vi "TestingBugFix.vi"() -> ()   [LabVIEW 2010]
uses:
  cm2nm_sample_set.ctl
  cm2nm_coordinate_information_v2.ctl
panel:
  out "Current Session Information":T1={"CollectionOfPoints"=[{"MetaDataFile"=path "", "X"=6.4684, "Y"=5.668, "Group"=0, "Z"=9.9998, "Rotation"=0.0, "Fiducial"=TRUE, "Magnification"=0.0, "Working_Distance"=0.0, "Notes"="Enter notes about this spot here.", "Location Name/ID"="Fid1", "OtherRelatedDataFiles"=[], "Available"=FALSE}, {"MetaDataFile"=path "", "X"=6.7812, "Y"=-3.8607, "Group"=0, "Z"=9.9998, "Rotation"=0.0, "Fiducial"=TRUE, "Magnification"=0.0, "Working_Distance"=0.0, "Notes"="Enter notes about this spot here.", "Location Name/ID"="Fid2", "OtherRelatedDataFiles"=[], "Available"=FALSE}, {"MetaDataFile"=path "", "X"=-3.5669, "Y"=-7.5774, "Group"=0, "Z"=9.9998, "Rotation"=0.0, "Fiducial"=TRUE, "Magnification"=0.0, "Working_Distance"=0.0, "Notes"="Enter notes about this spot here.", "Location Name/ID"="Fid3", "OtherRelatedDataFiles"=[], "Available"=FALSE}, {"MetaDataFile"=path "", "X"=4.04214894226502, "Y"=-0.78740272281952, "Group"=0, "Z"=9.9998, "Rotation"=0.0, "Fiducial"=FALSE, "Magnification"=0.0, "Working_Distance"=0.0, "Notes"="This is what we saw at the calculated coordinates for POI1. It's obviously not right! Look at images for calculated POI1.", "Location Name/ID"="POI1-calculated", "OtherRelatedDataFiles"=[], "Available"=FALSE}, {"MetaDataFile"=path "", "X"=0.4122, "Y"=-2.0241, "Group"=0, "Z"=0.0, "Rotation"=0.0, "Fiducial"=FALSE, "Magnification"=0.0, "Working_Distance"=0.0, "Notes"="These are the current coordinates of the real point", "Location Name/ID"="Actual POI1", "OtherRelatedDataFiles"=[], "Available"=FALSE}, {"MetaDataFile"=path "", "X"=0.41202447787402247, "Y"=-2.022580250416809, "Group"=20, "Z"=9.9998, "Rotation"=0.0, "Fiducial"=FALSE, "Magnification"=0.0, "Working_Distance"=0.0, "Notes"="Enter notes about this spot here.", "Location Name/ID"="POI1", "OtherRelatedDataFiles"=[], "Available"=FALSE}, {"MetaDataFile"=path "", "X"=-5.057894089920385, "Y"=8.260873627058263, "Group"=20, "Z"=9.9998, "Rotation"=0.0, "Fiducial"=TRUE, "Magnification"=0.0, "Working_Distance"=0.0, "Notes"="Enter notes about this spot here.", "Location Name/ID"="Fid5", "OtherRelatedDataFiles"=[], "Available"=FALSE}, {"MetaDataFile"=path "", "X"=-9.447460259107727, "Y"=0.8548991441777762, "Group"=20, "Z"=9.9998, "Rotation"=0.0, "Fiducial"=TRUE, "Magnification"=0.0, "Working_Distance"=0.0, "Notes"="Enter notes about this spot here.", "Location Name/ID"="Fid4", "OtherRelatedDataFiles"=[], "Available"=FALSE}], "Instrument"=0, "CollectionFile"=path "/INL Macintosh/Users/timothymcjunkin/Documents/First_round_samples_FY2011_Test/Sample_9 Karens Granite/Karens granite session 4 session5 session6/Session 5/Session 5.xml", "Session Name/ID"="Session 5", "SessionNotes"="This is what we saw at the calculated coordinates for POI1. It's obviously not right! Look at images for calculated POI1."} {"Instrument" items=["Unknown", "Phillips SEM IRC", "JEOL 7000F EML_MFC", "MXRD MFC", "JEOL_EPMA"]; "CollectionOfPoints"."Rotation" min=-37480660.29033894 max=37480660.27288565}
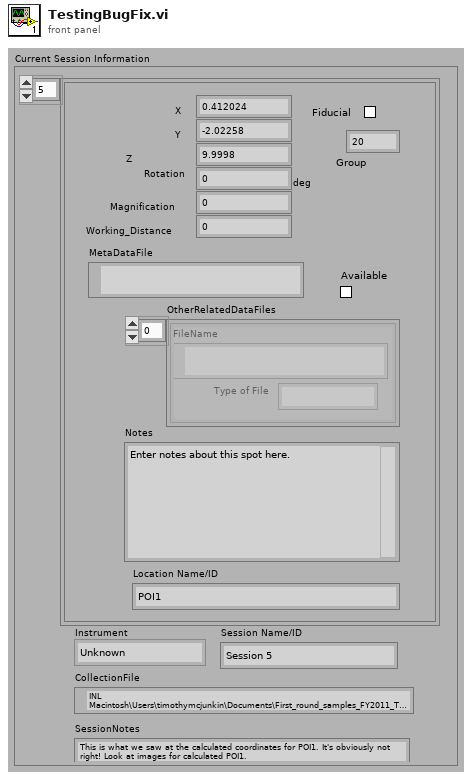
[diagram p1: front panel]
types:
  T1 = typedef "cm2nm_sample_set.ctl" = cluster{"CollectionOfPoints":T2[], "Instrument":u16, "CollectionFile":path, "Session Name/ID":string, "SessionNotes":string}
  T2 = typedef "cm2nm_coordinate_information_v2.ctl" = cluster{"MetaDataFile":path, "X":dbl, "Y":dbl, "Group":i32, "Z":dbl, "Rotation":dbl[unit], "Fiducial":bool, "Magnification":dbl, "Working_Distance":dbl, "Notes":string, "Location Name/ID":string, "OtherRelatedDataFiles":cluster{"Type of File":string, "FileName":path}[], "Available":bool}
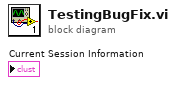
[diagram p0: block diagram]
diagram:
